vi "GCMPlugin_IsSupportingItem.vi"(8 "error in (no error)":errorcluster, 9 "VI Reference":refnum<vi>, 10 "ProjectItem Refnum":refnum<vi>, 11 "_ConnectorPaneEditor in":refnum<class "_ConnectorPaneEditor.lvclass">) -> (0 "error out":errorcluster, 2 "IsSupportingItem":bool, 3 "_ConnectorPaneEditor out":refnum<class "_ConnectorPaneEditor.lvclass">)   [LabVIEW 2014, in "_ConnectorPaneEditor.lvclass"]
uses:
  _ConnectorPaneEditor.lvclass
  GCMCore/Providers/Veritech_GCM/Support/Utilites/_ProjectItemsUtilities/_VIType.ctl
  GCMCore/Providers/Veritech_GCM/Support/Utilites/_ProjectItemsUtilities/_ProjectItemsUtilities.lvlib
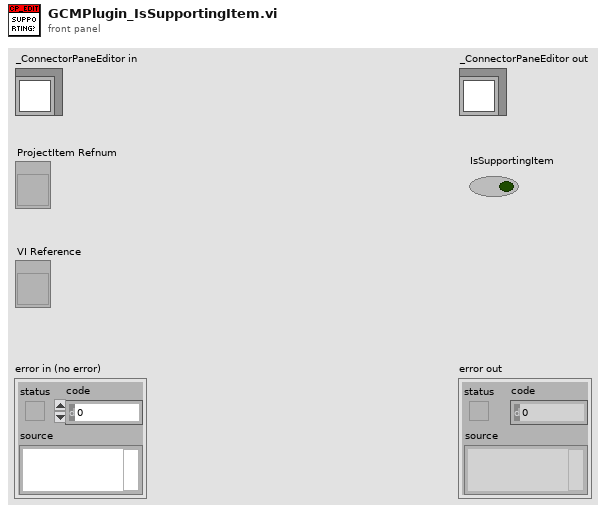
[diagram p1: front panel]
types:
  T1 = typedef "_ProjectItemsUtilities.lvlib/_VIType.ctl" = enum32{"invalid VI type", "Standard VI", "Control VI", "Global VI", "Polymorphic VI", "Configuration VI", "SubSystem", "Facade VI", "Method VI", "Statechart Diagram VI"}
  T2 = enum32{"invalid VI type", "Standard VI", "Control VI", "Global VI", "Polymorphic VI", "Configuration VI", "SubSystem", "Facade VI", "Method VI", "Statechart Diagram VI"}
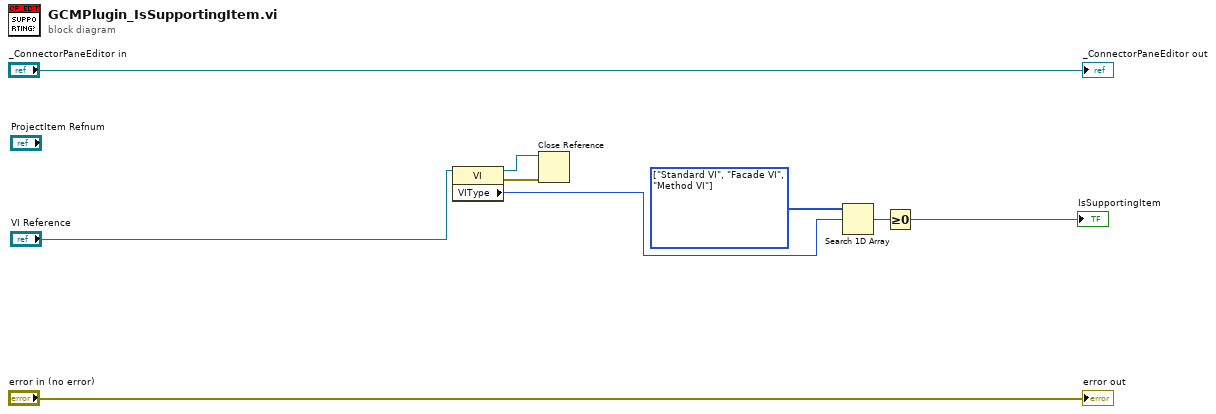
[diagram p0: block diagram]
diagram:
  w6 = T1[] [enum."Standard VI", enum."Facade VI", enum."Method VI"] items=["invalid VI type", "Standard VI", "Control VI", "Global VI", "Polymorphic VI", "Configuration VI", "SubSystem", "Facade VI", "Method VI", "Statechart Diagram VI"]
  n1 = property class="VI"(reference="VI Reference") -> (reference out=w3:refnum<vi>, error out=w4:errorcluster, "VIType"=w2:T2)  [unwired: 1 in]
  n2 = Close Reference(reference=w3, error in (no error)=w4) -> ()  [unwired: 1 out]
  n3 = Search 1D Array(1D array=w6, element=w2) -> (index of element=w5:i32)  [unwired: 1 in]
  n4 = Greater Or Equal To 0?(x=w5) -> (x >= 0?=→"IsSupportingItem":bool)
  "error out" <- "error in (no error)"
  "_ConnectorPaneEditor out" <- "_ConnectorPaneEditor in"
